vi "Detect Transition to TW.vi"(5 "Main References":T2, 8 "error in (no error)":errorcluster, 10 "Cart Array":bool[](array[boolean])) -> (0 "error out":errorcluster, 3 "Analysis":T1[](array[typedef]))   [LabVIEW 2018]
uses:
  Main Refs.ctl
  Hardware/Tecan/Pump Config.ctl
  Vacuum Specs.ctl
  Timing Specs.ctl
  Cartridges.ctl
  Cartridge Status.ctl
  Commands.ctl
  Lib/Time/Wells.ctl
  Lib/Time/Bottles.ctl
  Process State.ctl
  Vacuum Test.ctl
  Hardware/Mot Stage Mngr.ctl
  Hardware/Denkovi Mngr.ctl
  Hardware/DAQ Mngr.ctl
panel:
  # "Tecan Pump"
  # "Vacuum"
  # "General"
  # "Timing"
  # "Protocol"
  # "Zaber"
  # "NFC Reader 1"
  # "NFC  Reader 2"
  # "NFC Reader 3"
  # "NFC Reader 4"
  # "System"
  # "Cartridge Utitlies"
  # "Wells"
  # "times"
  # "from"
  # "State Machine"
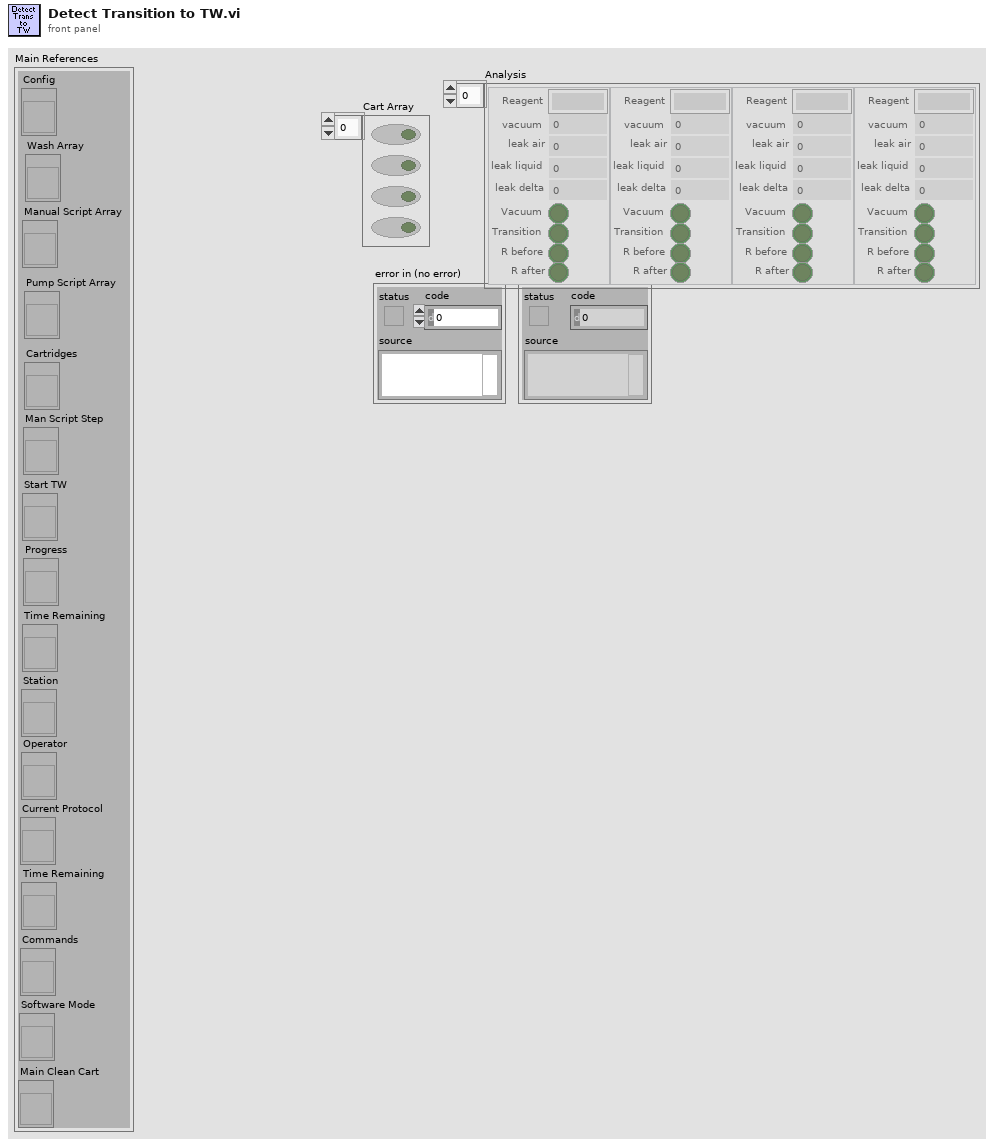
[diagram p1: front panel]
types:
  T1 = typedef "Vacuum Test.ctl" = cluster{"vacuum":dbl, "leak air":dbl, "leak liquid":dbl, "leak delta":dbl, "Transition":bool, "Vacuum":bool, "R before":bool, "R after":bool, "Reagent":string}
  T2 = typedef "Main Refs.ctl" = cluster{"Config":refnum<vi>, "Wash Array":refnum<vi>, "Manual Script Array":refnum<vi>, "Pump Script Array":refnum<vi>, "Cartridges":refnum<vi>, "Man Script Step":refnum<vi>, "Start TW":refnum<vi>, "Progress":refnum<vi>, "Time Remaining":refnum<vi>, "Station":refnum<vi>, "Operator":refnum<vi>, "Current Protocol":refnum<vi>, "Time Remaining":refnum<vi>, "Commands":refnum<vi>, "Software Mode":refnum<vi>, "Main Clean Cart":refnum<vi>}
  T3 = typedef "Denkovi Mngr.ctl" = enum16{"Init", "Set Peristaltic", "Set Vacuum", "Vac ON", "Vent&Close", "Set All Relays", "Set One Relay", "Read Relays", "Close"}
  T4 = typedef "DAQ Mngr.ctl" = enum16{"Init", "Read Vacuum", "Analyze Vacuum", "Read Cartridges", "Lock Cartridge", "Unlock Cartridge", "Read PS", "Close"}
  T5 = typedef "Mot Stage Mngr.ctl" = enum16{"Connect", "Init", "Status", "Send Cmd", "Current Pos", "Set Accel", "Set Max Vel", "Home", "Rel Move", "Abs Move", "Close"}
  T6 = typedef "Pump Config.ctl" = cluster{"Syringe size":u32, "Syringe address":u32, "# of ports":u32, "Init String":string, "Full Stroke (cnts)":i32, "Model":enum16{"XC", "Centris"}, "TW Position":dbl, "Load Position":dbl, "Bottom Position":dbl, "Station ID":string, "Vacuum Specs":T7, "Default Protocol":path, "Dry Time(s)":dbl, "Python Version":string, "NFC SN Array":string[], "Timing":T8}
  T7 = typedef "Vacuum Specs.ctl" = cluster{"vacuum max":dbl, "vacuum min":dbl, "liq2air rate delta":dbl, "liq2air time":dbl, "Conf. R":dbl, "LeakRateMax":dbl}
  T8 = typedef "Timing Specs.ctl" = cluster{"Checking vac and leak":dbl, "Priming input lines":dbl, "Rinsing syringe":dbl, "Filling well X w/ X":dbl, "Drain well X":dbl, "Clearing wells and lines":dbl, "Draining wells":dbl, "Rinsing all wells":dbl, "Testing for leaks/clogs":dbl, "Rinsing wells":dbl}
  T9 = typedef "Vacuum Output.ctl" = cluster{"Time(s)":dbl, "Vacuum":dbl, "Rate":dbl, "R":dbl}
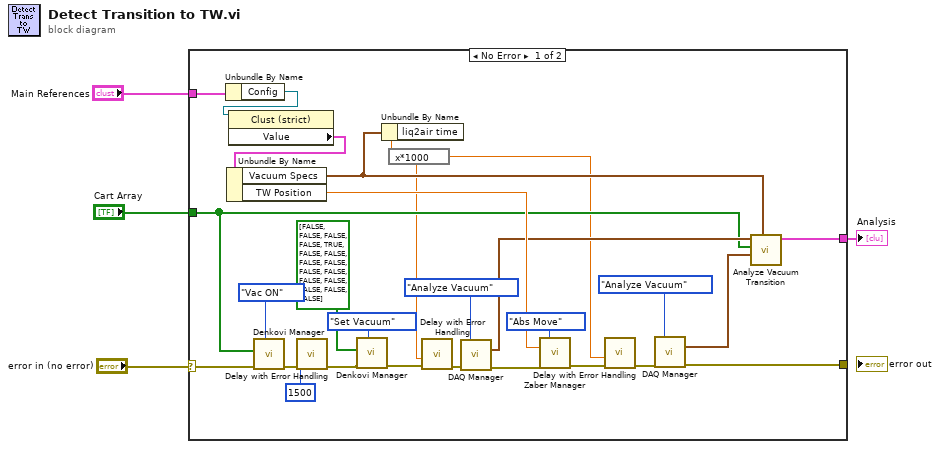
[diagram p0: block diagram]
diagram:
  n1 = case shown="No Error" "error in (no error)" {
    selector: "error in (no error)" -> [w25 w32]
    tunnel: [w16 w32] -> _
    tunnel: "Cart Array" -> [w14 _]
    tunnel: "Main References" -> [w29 _]
    tunnel: [w15 _] -> w4
    frame No Error {
      n2 = Unbundle By Name(w29) -> ("Config"=w31:refnum<vi>)
      n3 = property class="Clust (strict)"(reference=w31) -> ("Value"=w28:T6)  [unwired: 1 in, 2 out]
      n4 = Unbundle By Name(w28) -> ("Vacuum Specs"=w7:T7, "TW Position"=w27:dbl)
      n5 = call "Denkovi Manager.vi"("Action"=Denkovi_Mngr."Vac ON", "error in (no error)"=w25, "Relays In"=w14) -> ("error out"=w12:errorcluster)  [unwired: 6 in, 2 out]
      n6 = call "Delay with Error Handling.vi"("error in (no error)"=w12, "Delay (ms)"=u32 1500) -> ("error out"=w9:errorcluster)  [unwired: 9 in]
      n7 = call "Denkovi Manager.vi"("Action"=Denkovi_Mngr."Set Vacuum", "error in (no error)"=w9, "Relays In"=bool[] [FALSE, FALSE, FALSE, FALSE, TRUE, FALSE, FALSE, FALSE, FALSE, FALSE, FALSE, FALSE, FALSE, FALSE, FALSE, FALSE]) -> ("error out"=w8:errorcluster)  [unwired: 6 in, 2 out]
      n8 = Unbundle By Name(w7) -> ("liq2air time"=w6:dbl)
      n9 = expression code="x*1000"(w6) -> (w5:dbl)
      n10 = call "Delay with Error Handling.vi"("error in (no error)"=w8, "Delay (ms)"=w5) -> ("error out"=w24:errorcluster)  [unwired: 9 in]
      n11 = call "DAQ Manager.vi"("DAQ Mngr Action"=DAQ_Mngr."Analyze Vacuum", "error in (no error)"=w24) -> ("Data Array"=w18:T9[], "error out"=w23:errorcluster)  [unwired: 7 in, 5 out]
      n12 = call "Zaber Manager.vi"("Action"=Mot_Stage_Mngr."Abs Move", "Value"=w27, "error in (no error)"=w23) -> ("error out"=w21:errorcluster)  [unwired: 6 in, 6 out]
      n13 = call "Delay with Error Handling.vi"("error in (no error)"=w21, "Delay (ms)"=w5) -> ("error out"=w20:errorcluster)  [unwired: 9 in]
      n14 = call "DAQ Manager.vi"("DAQ Mngr Action"=DAQ_Mngr."Analyze Vacuum", "error in (no error)"=w20) -> ("Data Array"=w17:T9[], "error out"=w16:errorcluster)  [unwired: 7 in, 5 out]
      n15 = call "Analyze Vacuum Transition.vi"("Vacuum Specs"=w7, "Data After"=w17, "Cart Array"=w14, "Data Before"=w18) -> ("Analysis"=w15:T1[])  [unwired: 5 in, 2 out]
    }
    frame Error {
    }
  }
  "Analysis" <- w4
